vi "RT Host - new target.vi"(7 "Current Pos (mm)":dbl[](array[numeric]), 8 "error in":errorcluster, 11 "Target Pos (mm)":dbl[](array[numeric])) -> (0 "error out":errorcluster, 2 "Previous Target Pos (mm)":dbl[](array[numeric]), 3 "New Target?":bool)   [LabVIEW 2017]
doc: "This subVI compares the previous target position to the latest target position to see if it has changed. If it hasa Boolean TRUE value is outputted."
panel:
  # "Inputs"
  # "Outputs"
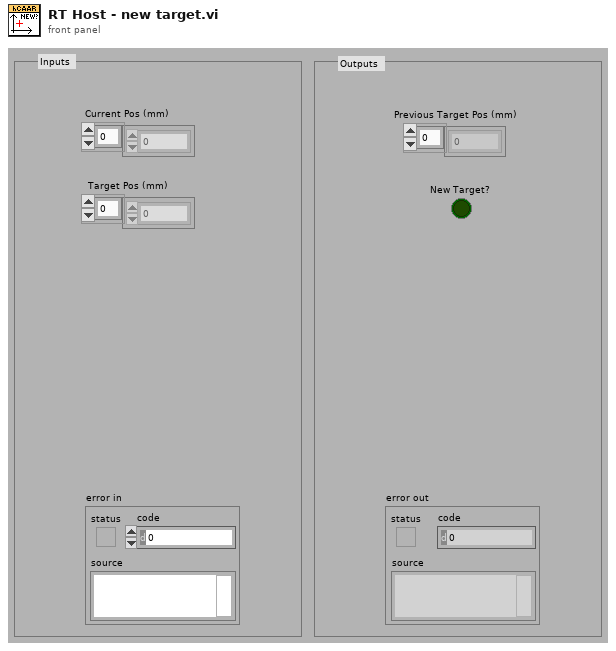
[diagram p1: front panel]
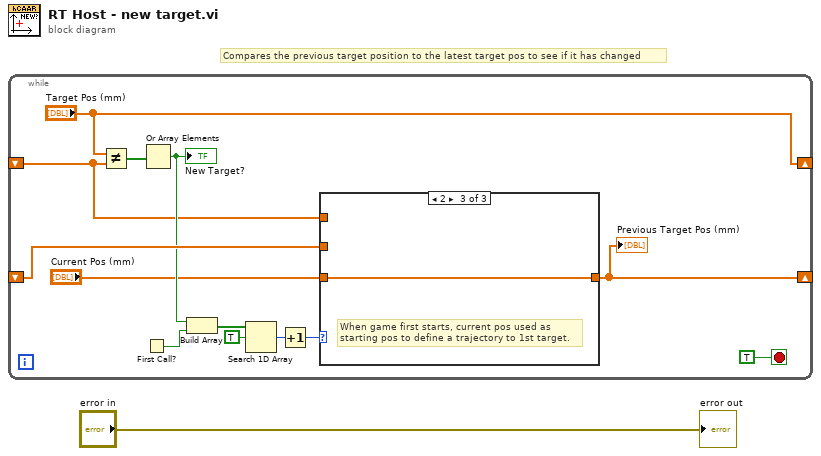
[diagram p0: block diagram]
diagram:
  # "Compares the previous target position to the latest target pos to see if it has changed"
  n1 = while {
    shift-right: [w4] -> _
    shift-left: _ -> [w7]
    shift-right: ["Target Pos (mm)"] -> _
    shift-left: _ -> [w2]
    stop <- TRUE stop-if-true
    n2 = Not Equal?(x="Target Pos (mm)", y=w2) -> (x != y?=w13:bool[])
    n3 = First Call?() -> (First Call?: T/F=w12:bool)
    n4 = Or Array Elements(Boolean array=w13) -> (logical OR=w6:bool)
    "New Target?" <- w6
    n5 = Build Array(w6, w12) -> (w11:bool[])
    n6 = Search 1D Array(1D array=w11, element=TRUE) -> (index of element=w9:i32)  [unwired: 1 in]
    n7 = Increment(x=w9) -> (x+1=w8:i32)
    n8 = case shown="2" w8 {
      tunnel: w2 -> [_ w16 _]
      tunnel: w7 -> [w15 _ _]
      tunnel: "Current Pos (mm)" -> [_ _ w17]
      tunnel: [w15 w16 w17] -> w4
      frame 0, Default {
        # "Previous target info sent round until\na new target is defined."
      }
      frame 1 {
        # "As a new target is added then the\nprevious target is sent to S-Register"
      }
      frame 2 {
        # "When game first starts, current pos used as\nstarting pos to define a trajectory to 1st target."
      }
    }
    "Previous Target Pos (mm)" <- w4
  }
  "error out" <- "error in"
